vi "Exploring data entry.vi"() -> ()   [LabVIEW 2015]
uses:
  <vilib>/Utility/miscctls.llb/LVRowAndColumnTypeDef.ctl
  <vilib>/Utility/miscctls.llb/LVBoundsTypeDef.ctl
  <vilib>/event_ctls.llb/eventvkey.ctl
panel:
  in  "Cancel":bool
  in  "Product":u16(ring) items=["Select...", "One", "Two", "Three", "Four"]
  in  "Week":enum8{"This Week", "Next Week"}(ring)=enum."Next Week"
  in  "Dilute":bool
  in  "Amount":dbl=10.0 min=0.0
  out "Table Indicator":string[][](table)=[["Select...", "0.00", "This Week", "0.0", "0", "0", "0", "0", "0", "0", "0", "0"], ["Select...", "0.00", "This Week", "0.0", "0", "0", "0", "0", "0", "0", "0", "0"], ["Select...", "0.00", "This Week", "0.0", "0", "0", "0", "0", "0", "0", "0", "0"], ["Select...", "0.00", "This Week", "0.0", "0", "0", "0", "0", "0", "0", "0", "0"], ["Select...", "0.00", "This Week", "0.0", "0", "0", "0", "0", "0", "0", "0", "0"], ["Select...", "0.00", "This Week", "0.0", "0", "0", "0", "0", "0", "0", "0", "0"], ["Select...", "0.00", "This Week", "0.0", "0", "0", "0", "0", "0", "0", "0", "0"], ["Select...", "0.00", "This Week", "0.0", "0", "0", "0", "0", "0", "0", "0", "0"], ["Select...", "0.00", "This Week", "0.0", "0", "0", "0", "0", "0", "0", "0", "0"], ["Select...", "0.00", "This Week", "0.0", "0", "0", "0", "0", "0", "0", "0", "0"], ["Total", "", "", "0", "0", "0", "0", "0", "0", "0", "0", ""]]
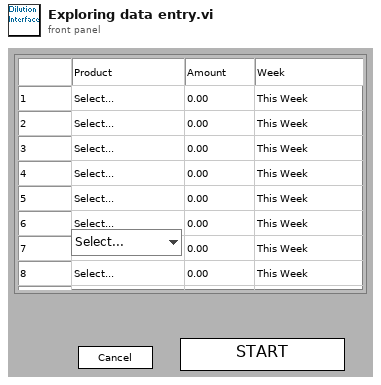
[diagram p1: front panel]
types:
  T1 = typedef "LVRowAndColumnTypeDef.ctl" = cluster{"Row":i32, "Column":i32}
  T2 = cluster{"Product":u16, "Amount":dbl, "Week":enum8{"This Week", "Next Week"}}
  T3 = cluster{"Product":u16, "Amount":dbl, "Week":enum8{"This Week", "Next Week"}}[]
  T4 = typedef "LVBoundsTypeDef.ctl" = cluster{"Width":u32, "Height":u32}
  T5 = typedef "eventvkey.ctl" = enum16{"ASCII", "Enter", "Return", "Shift", "Ctrl", "Alt", "Cmd", "Opt", "Caps", "NumLock", "Clear", "Break", "Up", "Down", "Left", "Right", "Insert", "Delete", "Home", "End", "PageUp", "PageDown", "Escape", "Help", "Pause", "ScrollLock", "F1", "F2", "F3", "F4", "F5", "F6", "F7", "F8", "F9", "F10", "F11", "F12", "F13", "F14", "F15", "F16", "F17", "F18", "F19", "F20", "F21", "F22", "F23", "F24", "Play", "VolumeUp", "VolumeDown", "Mute", "Two Byte Char"}
  T6 = typedef "LVPoint32TypeDef.ctl" = cluster{"Horizontal":i32, "Vertical":i32}
  T7 = typedef "LVPositionTypeDef.ctl" = cluster{"Left":i32, "Top":i32}
  T8 = typedef "LVFontTypeDef.ctl" = cluster{"Font Name":string, "Size":u16, "Bold":bool, "Italic":bool, "Underline":bool, "Strikeout":bool, "Color":u32}
  T9 = cluster{"Shift":bool, "Ctrl":bool, "Alt":bool, "Cmd":bool, "Opt":bool}
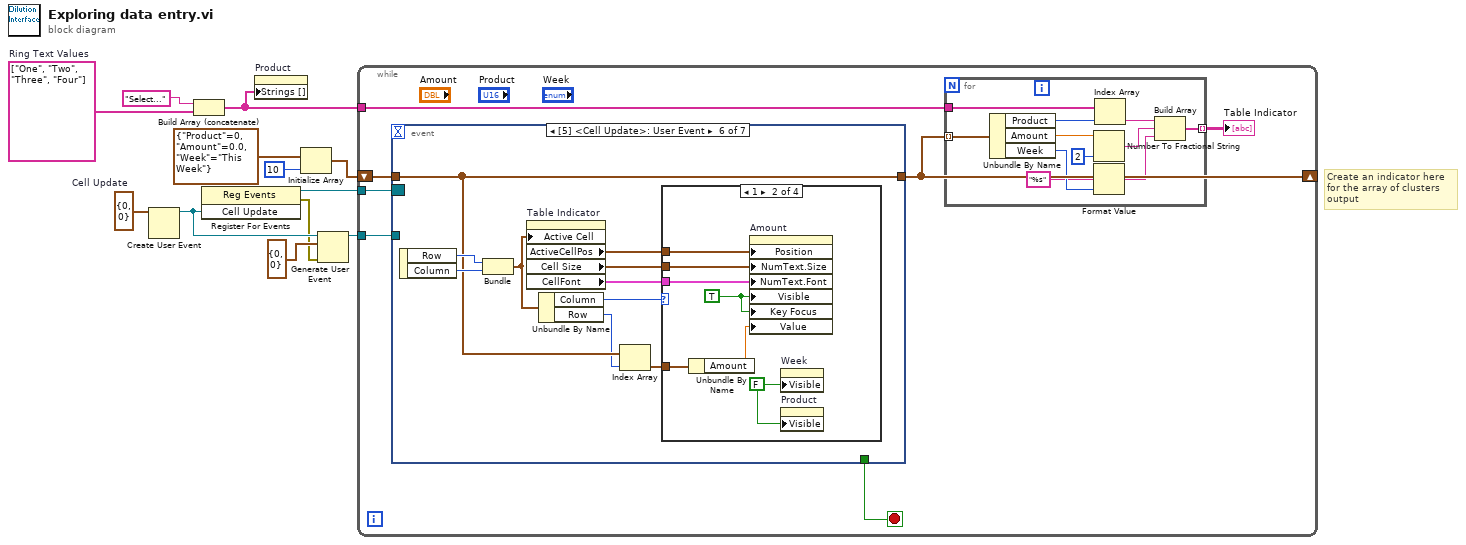
[diagram p0: block diagram]
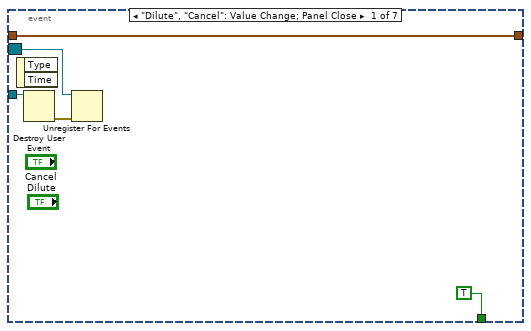
[diagram p2: hidden frame]
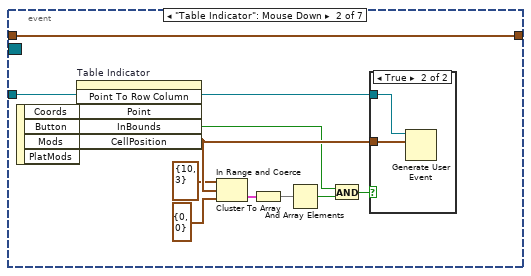
[diagram p3: hidden frame]
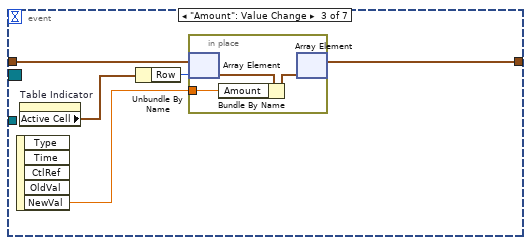
[diagram p5: hidden frame]
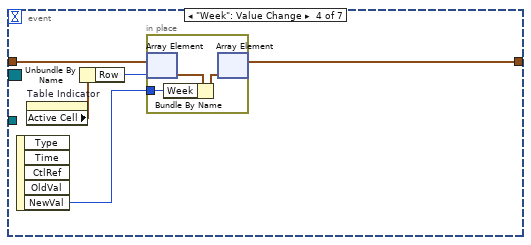
[diagram p6: hidden frame]
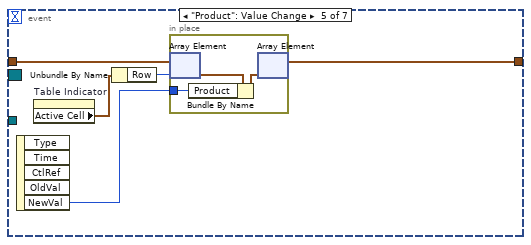
[diagram p7: hidden frame]
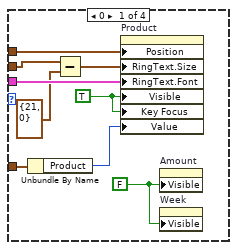
[diagram p8: hidden frame]
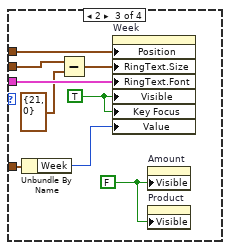
[diagram p9: hidden frame]
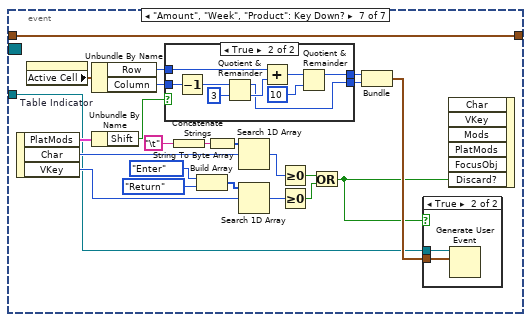
[diagram p11: hidden frame]
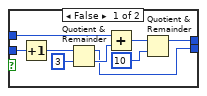
[diagram p13: hidden frame]
diagram:
  w1 = string[] ["One", "Two", "Three", "Four"]  # Ring Text Values
  w10 = T1 {"Row"=0, "Column"=0}  # Cell Update
  # "Create an indicator here\nfor the array of clusters\noutput"
  n1 = Create User Event(user event datatype=w10) -> (user event=w6:refnum<user-event>)  [unwired: 1 in, 1 out]
  n2 = Build Array (concatenate)("Select..." ("Product"), w1) -> (w2:string[])
  n3 = register-events(w6) -> (reference out=w9:refnum<event-registration>, error out=w4:errorcluster)  [unwired: 2 in]
  n4 = property on="Product" class="Ring (strict)"("Strings []"=w2) -> ()  [unwired: 2 in, 2 out]
  n5 = Initialize Array(T2 {"Product"=0, "Amount"=0.0, "Week"=enum."This Week"} ("Dilution Product Selection"), 10 ("dimension size")) -> (w11:T3)
  n6 = Generate User Event(user event=w6, event data cluster=T1 {"Row"=0, "Column"=0} ("event data"), error in=w4) -> (user event out=w3:refnum<user-event>)  [unwired: 1 in, 1 out]
  n7 = while {
    shift-right: [w16] -> _
    shift-left: w11 -> [w18]
    tunnel: w9 -> [w17]
    tunnel: w3 -> [w15]
    tunnel: w2 -> [w14]
    stop <- w19 stop-if-true
    n8 = event shown="[5] <Cell Update>: User Event" {
      selector: w17 -> [w32 _ _ _ _ _ _]
      dyn-events: _ -> [_ _ _ _ _ _ _]
      timeout: _ -> [_ _ _ _ _ _ _]
      tunnel: [TRUE ("Dilute") _ _ _ _ _ _] -> w19
      tunnel: w18 -> [w35 w37 w53 w61 w69 w75 w130]
      tunnel: [w35 w37 w51 w59 w67 w75 w130] -> w16
      tunnel: w15 -> [w33 w36 _ _ _ _ w108]
      event "Dilute", "Cancel": Value Change; Panel Close {
        n9 = event-data() -> ()  [unwired: 1 in, 2 out]
        n10 = Destroy User Event(user event=w33) -> (error out=w31:errorcluster)  [unwired: 1 in]
        n11 = Unregister For Events(event registration refnum=w32, error in=w31) -> ()  [unwired: 1 out]
      }
      event "Table Indicator": Mouse Down {
        n12 = event-data() -> ("Coords"=w46:T6)  [unwired: 1 in, 3 out]
        n13 = invoke on="Table Indicator" class="Tbl (strict)" method="Point To Row Column"("Point"=w46) -> ("InBounds"=w41:bool, "CellPosition"=w45:T1)  [unwired: 5 in, 4 out]
        n14 = In Range and Coerce(upper limit=T1 {"Row"=10, "Column"=3}, x=w45, lower limit=T1 {"Row"=0, "Column"=0}) -> (In Range?=w42:cluster{"Row":bool, "Column":bool})  [unwired: 1 out]
        n15 = Cluster To Array(cluster=w42) -> (array=w39:bool[])
        n16 = And Array Elements(Boolean array=w39) -> (logical AND=w38:bool)
        n17 = And(x=w41, y=w38) -> (x .and. y?=w40:bool)
        n18 = case shown="True" w40 {
          tunnel: w45 -> [_ w48]
          tunnel: w36 -> [_ w47]
          frame False {
          }
          frame True {
            n19 = Generate User Event(user event=w47, event data cluster=w48) -> ()  [unwired: 2 in, 2 out]
          }
        }
      }
      event "Amount": Value Change {
        n20 = event-data() -> ("NewVal"=w50:dbl)  [unwired: 1 in, 4 out]
        n21 = property on="Table Indicator" class="Tbl (strict)"() -> ("Active Cell"=w49:T1)  [unwired: 2 in, 2 out]
        n22 = Unbundle By Name(w49) -> ("Row"=w52:i32)
        n23 = in-place {
          in-place-border: w50 -> [w54]
          n24 = in-place-array #1(w53, w52) -> (w56:T2)
          n25 = Bundle By Name(cluster=w56, "Amount"=w54) -> (w55:T2)
          n26 = in-place-array #1(w55) -> (w51:T3)  [unwired: 1 out]
        }
      }
      event "Week": Value Change {
        n27 = event-data() -> ("NewVal"=w58:enum8{"This Week", "Next Week"})  [unwired: 1 in, 4 out]
        n28 = property on="Table Indicator" class="Tbl (strict)"() -> ("Active Cell"=w57:T1)  [unwired: 2 in, 2 out]
        n29 = Unbundle By Name(w57) -> ("Row"=w60:i32)
        n30 = in-place {
          in-place-border: w58 -> [w62]
          n31 = in-place-array #2(w61, w60) -> (w64:T2)
          n32 = Bundle By Name(cluster=w64, "Week"=w62) -> (w63:T2)
          n33 = in-place-array #2(w63) -> (w59:T3)  [unwired: 1 out]
        }
      }
      event "Product": Value Change {
        n34 = event-data() -> ("NewVal"=w66:u16)  [unwired: 1 in, 4 out]
        n35 = property on="Table Indicator" class="Tbl (strict)"() -> ("Active Cell"=w65:T1)  [unwired: 2 in, 2 out]
        n36 = Unbundle By Name(w65) -> ("Row"=w68:i32)
        n37 = in-place {
          in-place-border: w66 -> [w70]
          n38 = in-place-array #3(w69, w68) -> (w72:T2)
          n39 = Bundle By Name(cluster=w72, "Product"=w70) -> (w71:T2)
          n40 = in-place-array #3(w71) -> (w67:T3)  [unwired: 1 out]
        }
      }
      event User Event {
        n41 = event-data() -> ("Row"=w82:i32, "Column"=w81:i32)  [unwired: 1 in]
        n42 = Bundle("Row"=w82, "Column"=w81) -> (w76:cluster{"Row":i32, "Column":i32})  [unwired: 1 in]
        n43 = property on="Table Indicator" class="Tbl (strict)"("Active Cell"=w76) -> ("ActiveCellPos"=w80:T7, "Cell Size"=w79:T4, "CellFont"=w77:T8)  [unwired: 2 in, 2 out]
        n44 = Unbundle By Name(w76) -> ("Column"=w78:i32, "Row"=w74:i32)
        n45 = Index Array(array=w75, index=w74) -> (element=w73:T2)
        n46 = case shown="1" w78 {
          tunnel: w80 -> [w91 w98 w107 _]
          tunnel: w79 -> [w85 w97 w106 _]
          tunnel: w77 -> [w89 w94 w104 _]
          tunnel: w73 -> [w84 w93 w99 _]
          frame 0 {
            w90 = FALSE ("Visible")
            w88 = TRUE ("Key Focus")
            n47 = Unbundle By Name(w84) -> ("Product"=w83:u16)
            n48 = Subtract(x=w85, y=T4 {"Width"=21, "Height"=0} ("x")) -> (x-y=w86:T4)
            n49 = property on="Product" class="Ring (strict)"("Position"=w91, "RingText.Size"=w86, "RingText.Font"=w89, "Visible"=w88, "Key Focus"=w88, "Value"=w83) -> ()  [unwired: 2 in, 2 out]
            n50 = property on="Amount" class="DigNum (strict)"("Visible"=w90) -> ()  [unwired: 2 in, 2 out]
            n51 = property on="Week" class="Enum (strict)"("Visible"=w90) -> ()  [unwired: 2 in, 2 out]
          }
          frame 1 {
            w96 = FALSE ("Visible")
            w95 = TRUE ("Key Focus")
            n52 = Unbundle By Name(w93) -> ("Amount"=w92:dbl)
            n53 = property on="Amount" class="DigNum (strict)"("Position"=w98, "NumText.Size"=w97, "NumText.Font"=w94, "Visible"=w95, "Key Focus"=w95, "Value"=w92) -> ()  [unwired: 2 in, 2 out]
            n54 = property on="Week" class="Enum (strict)"("Visible"=w96) -> ()  [unwired: 2 in, 2 out]
            n55 = property on="Product" class="Ring (strict)"("Visible"=w96) -> ()  [unwired: 2 in, 2 out]
          }
          frame 2 {
            w105 = FALSE ("Visible")
            w103 = TRUE ("Key Focus")
            n56 = Unbundle By Name(w99) -> ("Week"=w100:enum8{"This Week", "Next Week"})
            n57 = Subtract(x=w106, y=T4 {"Width"=21, "Height"=0} ("x")) -> (x-y=w102:T4)
            n58 = property on="Week" class="Enum (strict)"("Position"=w107, "RingText.Size"=w102, "RingText.Font"=w104, "Visible"=w103, "Key Focus"=w103, "Value"=w100) -> ()  [unwired: 2 in, 2 out]
            n59 = property on="Amount" class="DigNum (strict)"("Visible"=w105) -> ()  [unwired: 2 in, 2 out]
            n60 = property on="Product" class="Ring (strict)"("Visible"=w105) -> ()  [unwired: 2 in, 2 out]
          }
          frame Default {
          }
        }
      }
      event "Amount", "Week", "Product": Key Down? {
        n61 = event-data() -> ("PlatMods"=w109:T9, "Char"=w117:i16, "VKey"=w113:T5)  [unwired: 1 in]
        n62 = property on="Table Indicator" class="Tbl (strict)"() -> ("Active Cell"=w123:T1)  [unwired: 2 in, 2 out]
        n63 = Unbundle By Name(w123) -> ("Row"=w128:i32, "Column"=w129:i32)
        n64 = Unbundle By Name(w109) -> ("Shift"=w124:bool)
        n65 = case shown="True" w124 {
          tunnel: w129 -> [w141 w150]
          tunnel: w128 -> [w137 w146]
          tunnel: [w134 w143] -> w127
          tunnel: [w133 w142] -> w126
          frame False {
            n66 = Increment(x=w141) -> (x+1=w140:i32)
            n67 = Quotient & Remainder(x=w140, y=3) -> (x-y*floor(x/y)=w133:i32, floor(x/y)=w138:i32)
            n68 = Add(x=w137, y=w138) -> (x+y=w136:i32)
            n69 = Quotient & Remainder(x=w136, y=10) -> (x-y*floor(x/y)=w134:i32)  [unwired: 1 out]
          }
          frame True {
            n70 = Decrement(x=w150) -> (x-1=w149:i32)
            n71 = Quotient & Remainder(x=w149, y=3) -> (x-y*floor(x/y)=w142:i32, floor(x/y)=w147:i32)
            n72 = Add(x=w146, y=w147) -> (x+y=w145:i32)
            n73 = Quotient & Remainder(x=w145, y=10) -> (x-y*floor(x/y)=w143:i32)  [unwired: 1 out]
          }
        }
        n74 = Concatenate Strings("\t") -> (w121:string)
        n75 = Build Array(eventvkey."Enter" ("VKey"), eventvkey."Return" ("VKey")) -> (w114:T5[])
        n76 = String To Byte Array(string=w121) -> (unsigned byte array=w120:u8[])
        n77 = Search 1D Array(1D array=w120, element=w117) -> (index of element=w119:i32)  [unwired: 1 in]
        n78 = Search 1D Array(1D array=w114, element=w113) -> (index of element=w112:i32)  [unwired: 1 in]
        n79 = Greater Or Equal To 0?(x=w119) -> (x >= 0?=w118:bool)
        n80 = Greater Or Equal To 0?(x=w112) -> (x >= 0?=w110:bool)
        n81 = Or(x=w118, y=w110) -> (x .or. y?=w111:bool)
        n82 = Bundle(w127, w126) -> (w125:cluster{i32, i32})  [unwired: 1 in]
        n83 = case shown="True" w111 {
          tunnel: w125 -> [_ w132]
          tunnel: w108 -> [_ w131]
          frame False {
          }
          frame True {
            n84 = Generate User Event(user event=w131, event data cluster=w132) -> ()  [unwired: 2 in, 2 out]
          }
        }
        n85 = event-data("Discard?"=w111) -> ()  [unwired: 6 in, 1 out]
      }
    }
    n86 = for {
      tunnel: [w24] -> w13 mode=indexing
      tunnel: w16 -> [w23] mode=indexing
      tunnel: w14 -> [w21]
      n87 = Unbundle By Name(w23) -> ("Product"=w20:u16, "Amount"=w27:dbl, "Week"=w30:enum8{"This Week", "Next Week"})
      n88 = Number To Fractional String(number=w27, precision (6)=i16 2) -> (F-format string=w26:string)  [unwired: 2 in]
      n89 = Format Value(format string="%s", value (0)=w30) -> (output string=w28:string)  [unwired: 1 in]
      n90 = Index Array(array=w21, index=w20) -> (element=w22:string)
      n91 = Build Array(w22, w26, w28) -> (w24:string[])
    }
    "Table Indicator" <- w13
  }
